vi "Periodic Tasks.vi"(8 "error in":errorcluster) -> ()   [LabVIEW 2019]
doc: "This VI runs in parallel to other tasks. It can contain as many user-defined periodic loops as you need. These can carry out PID or other sorts of timed response."
uses:
  <vilib>/Rock Robotics/WPI/Utilities/WPI_GetSetVariantRefNum.vi
  Robot Global Data.vi
  <vilib>/Rock Robotics/Network Tables/NT Read Number.vi
  <vilib>/Rock Robotics/WPI/RobotDrive/WPI_RobotDriveArcadeDrive_Standard(NoSaturation).vi
  <vilib>/Rock Robotics/Network Tables/NT Read Boolean.vi
panel:
  in  "Proportional Gain":dbl
  in  "Target X":dbl
  out "output":T1
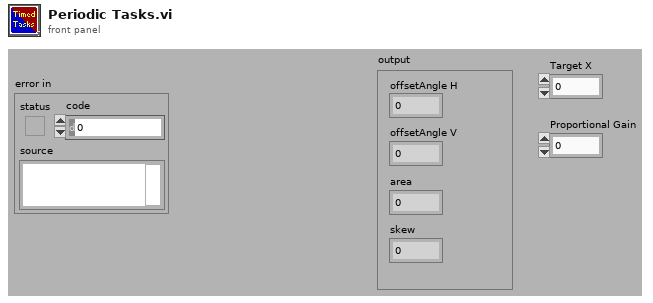
[diagram p1: front panel]
types:
  T1 = cluster{"offsetAngle H":dbl, "offsetAngle V":dbl, "area":dbl, "skew":dbl}
  T2 = typedef "WPI_JoystickDevRef.ctl" = cluster{"Device":T3}
  T3 = typedef "WPI_JoystickDeviceEnum.ctl" = enum16{"USB 0", "USB 1", "USB 2", "USB 3", "USB 4", "USB 5"}
  T4 = typedef "WPI_RobotDriveDevRef.ctl" = cluster{"DevStatus":errorcluster, "Motors[]":T5[], "Square Inputs":bool, "Max Output":dbl}
  T5 = typedef "WPI_MotorControlDeviceRef.ctl" = cluster{"DeviceStatus":errorcluster, "Type":T6, "PWM":cluster{"PWM Channel":T7, "DeadBand":T8}, "CAN":cluster{"Device Number":u8, "SetOutput VI Ref":variant, "GetOutput VI Ref":variant, "Enable VI Ref":variant, "Disable VI Ref":variant, "Data":variant}, "Invert":bool, "DIO PWM":cluster{"PWM \"Enable\" Channel":T7, "DIOChannel":T9, "PWM Rate":dbl}}
  T6 = typedef "WPI_MotorControlType.ctl" = enum16{"PWM", "CAN", "DIO PWM"}
  T7 = typedef "FPGA_DIOPWMChannel.ctl" = enum8{"PWM 0", "PWM 1", "PWM 2", "PWM 3", "PWM 4", "PWM 5", "PWM 6", "PWM 7", "PWM 8", "PWM 9", "PWM MXP 0", "PWM MXP 1", "PWM MXP 2", "PWM MXP 3", "PWM MXP 4", "PWM MXP 5", "PWM MXP 6", "PWM MXP 7", "PWM MXP 8", "PWM MXP 9", "Invalid"}
  T8 = typedef "WPI_PWMDeadband.ctl" = cluster{"Name":string, "maxPositivePwm":i32, "minPositivePwm":i32, "centerPwm":i32, "maxNegativePwm":i32, "minNegativePwm":i32, "angularRange":u16}
  T9 = typedef "FPGA_DIOChannel.ctl" = enum8{"DIO 0", "DIO 1", "DIO 2", "DIO 3", "DIO 4", "DIO 5", "DIO 6", "DIO 7", "DIO 8", "DIO 9", "DIO MXP 0", "DIO MXP 1", "DIO MXP 2", "DIO MXP 3", "DIO MXP 4", "DIO MXP 5", "DIO MXP 6", "DIO MXP 7", "DIO MXP 8", "DIO MXP 9", "DIO MXP 10", "DIO MXP 11", "DIO MXP 12", "DIO MXP 13", "DIO MXP 14", "DIO MXP 15", "SPI Port CS1", "SPI Port CS2", "SPI Port CS3", "SPI Port MISO", "SPI Port MOSI", "Invalid"}
  T10 = cluster{"JoystickDevRef":T2, "RobotDriveDevRef":T4}
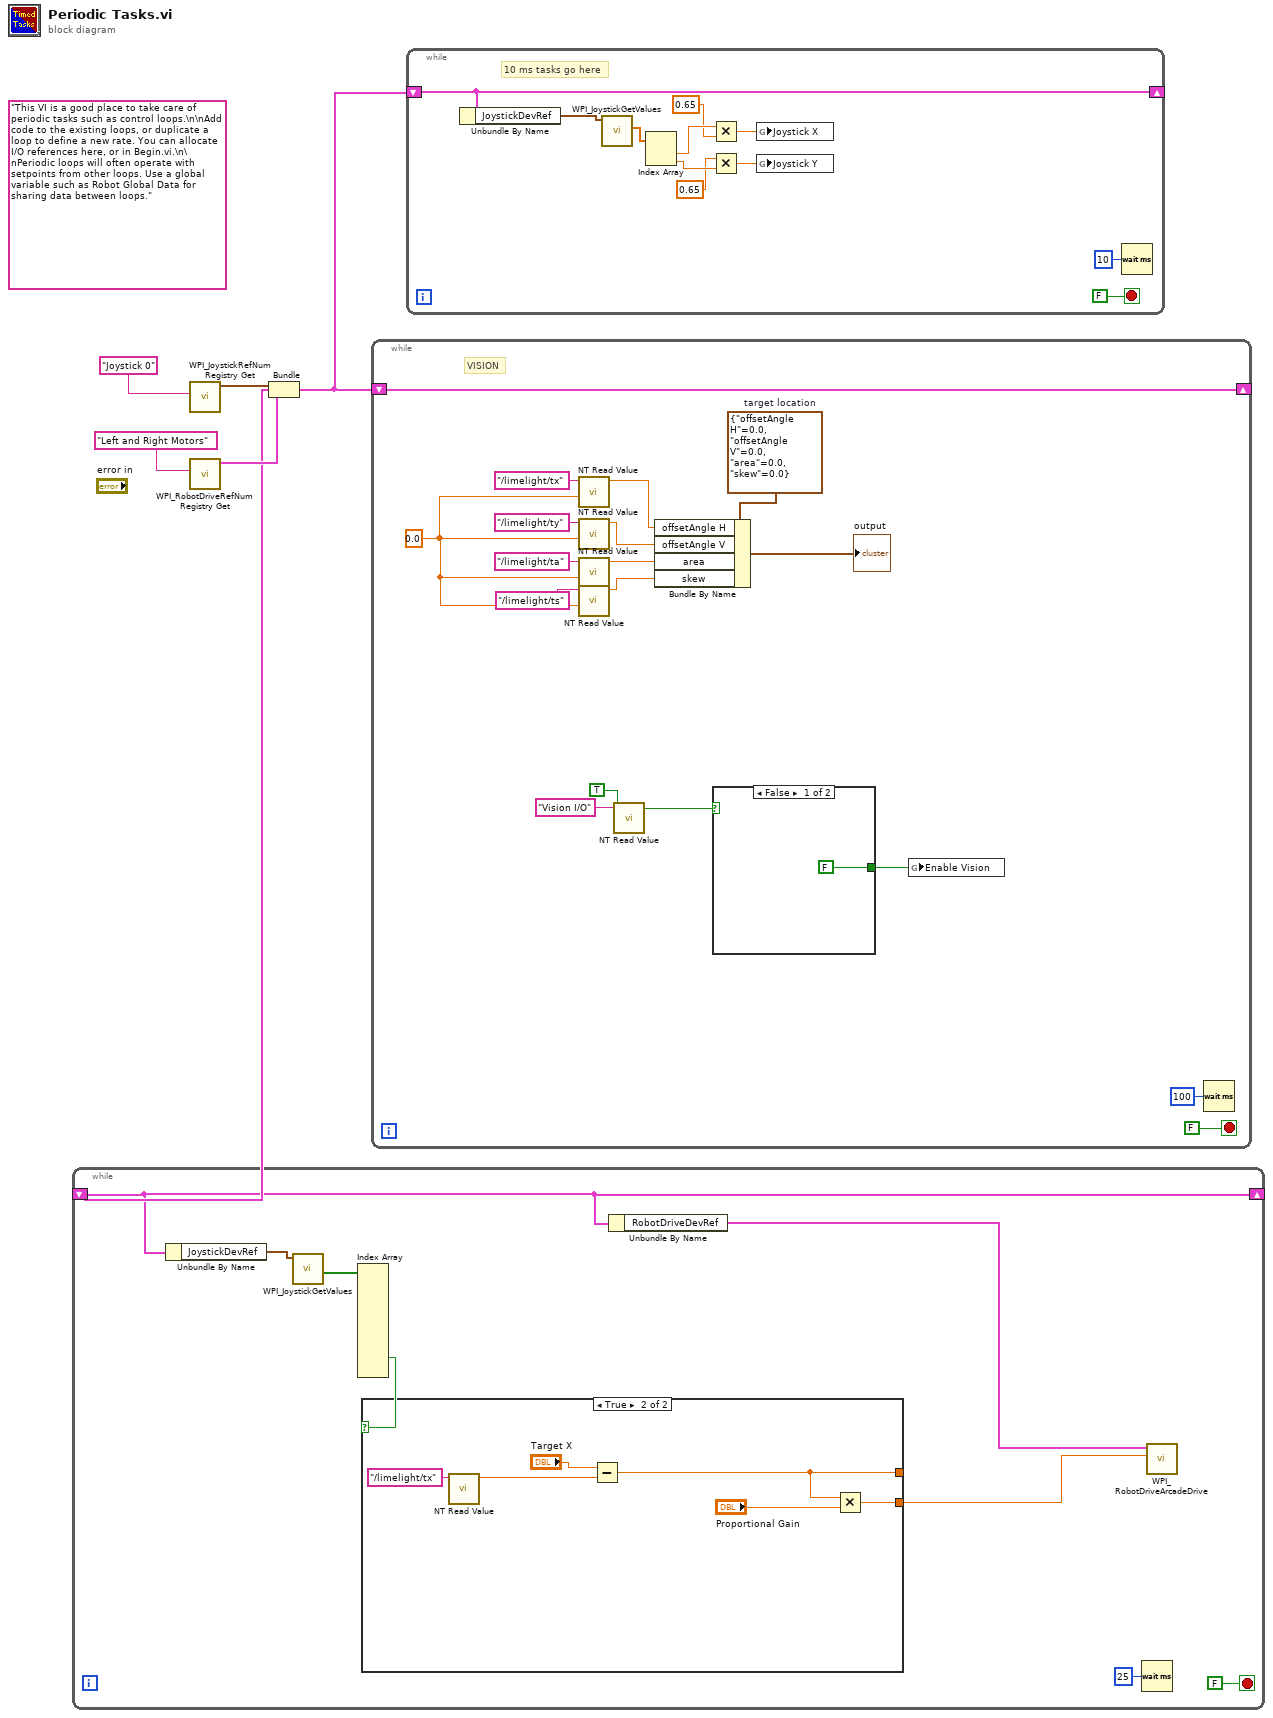
[diagram p0: block diagram]
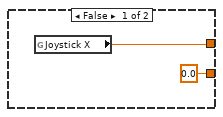
[diagram p2: hidden frame]
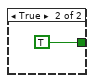
[diagram p3: hidden frame]
diagram:
  (unwired) "This VI is a good place to take care of periodic tasks such as control loops.\n\nAdd code to the existing loops, or duplicate a loop to define a new rate. You can allocate I/O references here, or in Begin.vi.\n\nPeriodic loops will often operate with setpoints from other loops. Use a global variable such as Robot Global Data for sharing data between loops."
  n1 = call <vilib>:"WPI_JoystickRefNum Registry Get.vi"("refnum name"="Joystick 0") -> ("JoystickDevRef"=w3:T2)  [unwired: 1 in, 9 out]
  n2 = call <vilib>:"WPI_RobotDriveRefNum Registry Get.vi"("refnum name"="Left and Right Motors") -> ("RobotDriveDevRef"=w2:T4)  [unwired: 1 in, 9 out]
  n3 = Bundle("JoystickDevRef"=w3, "RobotDriveDevRef"=w2) -> (w1:T10)  [unwired: 1 out]
  n4 = while {
    shift-right: [w11] -> _
    shift-left: w1 -> [w11]
    stop <- FALSE stop-if-true
    n5 = Unbundle By Name(w11) -> ("JoystickDevRef"=w10:T2)
    n6 = call <vilib>:"WPI_JoystickGetValues.vi"("JoystickDevRef"=w10) -> ("Buttons"=w9:bool[])  [unwired: 6 in, 4 out]
    n7 = Index Array(array=w9) -> (element #10=w8:bool)  [unwired: 12 in, 11 out]
    n8 = case shown="True" w8 {
      tunnel: [w15 w17] -> _
      tunnel: [0.0 w16] -> w6
      frame False {
        n9 = global read "Robot Global Data.vi" "Joystick X"() -> (w15:dbl)
      }
      frame True {
        n10 = call-poly <vilib>:"NT Read Value.vi"("Name"="/limelight/tx") -> ("Numeric"=w20:dbl)  [unwired: 9 in, 1 out]
        n11 = Subtract(x="Target X", y=w20) -> (x-y=w17:dbl)
        n12 = Multiply(x=w17, y="Proportional Gain") -> (x*y=w16:dbl)
      }
    }
    n13 = Unbundle By Name(w11) -> ("RobotDriveDevRef"=w7:T4)
    n14 = Wait (ms)(milliseconds to wait=u32 25) -> ()  [unwired: 1 out]
    n15 = call-poly <vilib>:"WPI_RobotDriveArcadeDrive.vi"("X axis value"=w6, "RobotDriveDevRef"=w7) -> ()  [unwired: 7 in, 3 out]
  }
  n16 = while {
    shift-right: [w26] -> _
    shift-left: w1 -> [w26]
    stop <- FALSE stop-if-true
    w27 = 0.0
    w36 = T1 {"offsetAngle H"=0.0, "offsetAngle V"=0.0, "area"=0.0, "skew"=0.0}  # target location
    # "VISION"
    n17 = call-poly <vilib>:"NT Read Value.vi"("Default Value"=w27, "Name"="/limelight/tx") -> ("Numeric"=w32:dbl)  [unwired: 8 in, 1 out]
    n18 = call-poly <vilib>:"NT Read Value.vi"("Default Value"=w27, "Name"="/limelight/ty") -> ("Numeric"=w33:dbl)  [unwired: 8 in, 1 out]
    n19 = call-poly <vilib>:"NT Read Value.vi"("Default Value"=w27, "Name"="/limelight/ta") -> ("Numeric"=w34:dbl)  [unwired: 8 in, 1 out]
    n20 = call-poly <vilib>:"NT Read Value.vi"("Default Value"=w27, "Name"="/limelight/ts") -> ("Numeric"=w35:dbl)  [unwired: 8 in, 1 out]
    n21 = call-poly <vilib>:"NT Read Value.vi"("Default Value"=TRUE, "Name"="Vision I/O") -> ("Boolean"=w23:bool)  [unwired: 8 in, 1 out]
    n22 = Bundle By Name(cluster=w36, "offsetAngle H"=w32, "offsetAngle V"=w33, "area"=w34, "skew"=w35) -> (→"output":T1)
    n23 = case shown="False" w23 {
      tunnel: [FALSE ("Enable Vision") TRUE ("Enable Vision")] -> w22
      frame False {
      }
      frame True {
      }
    }
    n24 = global write "Robot Global Data.vi" "Enable Vision"(w22) -> ()
    n25 = Wait (ms)(milliseconds to wait=u32 100) -> ()  [unwired: 1 out]
  }
  n26 = while {
    shift-right: [w50] -> _
    shift-left: w1 -> [w50]
    stop <- FALSE stop-if-true
    # "10 ms tasks go here"
    n27 = Unbundle By Name(w50) -> ("JoystickDevRef"=w49:T2)
    n28 = call <vilib>:"WPI_JoystickGetValues.vi"("JoystickDevRef"=w49) -> ("Axes"=w48:dbl[])  [unwired: 6 in, 4 out]
    n29 = Index Array(array=w48) -> (element #1=w47:dbl, element #2=w45:dbl)  [unwired: 2 in]
    n30 = Multiply(x=w47, y=0.65) -> (x*y=w43:dbl)
    n31 = Multiply(x=0.65, y=w45) -> (x*y=w42:dbl)
    n32 = global write "Robot Global Data.vi" "Joystick X"(w43) -> ()
    n33 = global write "Robot Global Data.vi" "Joystick Y"(w42) -> ()
    n34 = Wait (ms)(milliseconds to wait=u32 10) -> ()  [unwired: 1 out]
  }
